vi "Interpolate Arm System.vi"(8 "Duration":dbl, 9 "Current Time":dbl, 10 "Start Arm Motor Commands":T1, 11 "End Arm Motor Commands":T1) -> (3 "Current Arm Motor Commands":T1)   [LabVIEW 2018]
uses:
  Controls/Arm Motor Commands.ctl
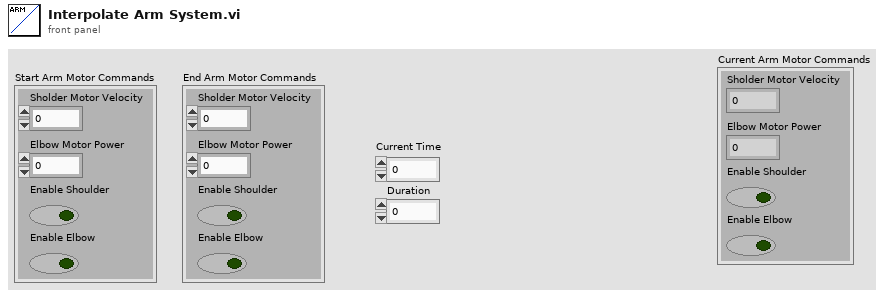
[diagram p1: front panel]
types:
  T1 = typedef "Arm Motor Commands.ctl" = cluster{"Enable Shoulder":bool, "Enable Elbow":bool, "Elbow Motor Power":dbl, "Sholder Motor Velocity":dbl}
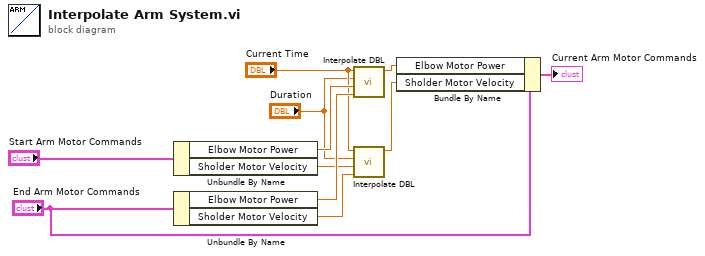
[diagram p0: block diagram]
diagram:
  n1 = Unbundle By Name("Start Arm Motor Commands") -> ("Elbow Motor Power"=w11:dbl, "Sholder Motor Velocity"=w5:dbl)
  n2 = Unbundle By Name("End Arm Motor Commands") -> ("Elbow Motor Power"=w10:dbl, "Sholder Motor Velocity"=w4:dbl)
  n3 = call "Interpolate DBL.vi"("Ending Value"=w10, "Starting Value"=w11, "Duration"="Duration", "Current Time"="Current Time") -> ("Current Value"=w9:dbl)  [unwired: 7 in]
  n4 = call "Interpolate DBL.vi"("Ending Value"=w4, "Starting Value"=w5, "Duration"="Duration", "Current Time"="Current Time") -> ("Current Value"=w1:dbl)  [unwired: 7 in]
  n5 = Bundle By Name(cluster="End Arm Motor Commands", "Elbow Motor Power"=w9, "Sholder Motor Velocity"=w1) -> (→"Current Arm Motor Commands":T1)
